vi "Iterator.vi"(8 "error in":errorcluster, 11 "Iterator Actor in":refnum<class "Abstract Iterator Actor.lvclass">) -> (0 "error out":errorcluster, 3 "Iterator Actor out":refnum<class "Abstract Iterator Actor.lvclass">)   [LabVIEW 2023, in "Iterator Actor.lvlib" / "Abstract Iterator Actor.lvclass"]
doc: "(<B>Filename</B>: Actor Framework.lvlib:Actor.lvclass:Actor Core.vi)\n\nReceives messages to the actor, reacts to them, and initiates any error handling that may shut the actor down.\n\nDescendant classes may override this VI to append parallel tasks for the actor to complete while it handles messages. Overrides use the Call Parent Method node."
uses:
  Abstract Iterator Actor.lvclass
  Abstract Iterator Actor.lvclass/Abstract Iterator Actor.ctl
  <vilib>/ActorFramework/Actor/Actor.lvclass/Actor.ctl
  <vilib>/ActorFramework/Message Enqueuer/Message Enqueuer.lvclass/Message Enqueuer.ctl
  Stop Reason.ctl
  <vilib>/ActorFramework/Message Enqueuer/Init from Existing Queue.vi
  <vilib>/ActorFramework/Message Enqueuer/Message Enqueuer.lvclass
  <vilib>/ActorFramework/Actor/Actor.lvclass
  Iterator Actor/Iterator Actor Messages/Report Iterations End Msg/Report Iterations End Msg.lvclass
  Iterator Actor/Iterator Actor Messages/Write Stop Reason Msg/Write Stop Reason Msg.lvclass
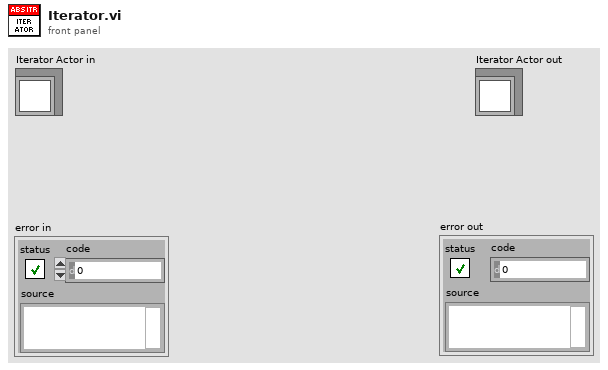
[diagram p1: front panel]
types:
  T1 = typedef "Iterator Actor.lvlib/Abstract Iterator Actor.lvclass/Iterator Settings.ctl" = cluster{"Prepare timeout (ms)":i32, "Iterate timeout (ms)":i32, "Conclude timeout (ms)":i32, "Iterate period (ms)":i32, "Number of iterations":i32, "Time before stop (ms)":i32, "Active Stop Conditions":T2, "Prepare Msg":refnum<class "Message.lvclass">, "Iterate Msg":refnum<class "Message.lvclass">, "Conclude Msg":refnum<class "Message.lvclass">, "Iterations End Report":refnum<class "Iterator Report Iterations End Msg.lvclass">}
  T2 = typedef "Iterator Actor.lvlib/Abstract Iterator Actor.lvclass/Active Stop Conditions.ctl" = cluster{"Number of Iterations":bool, "Time Elapsed":bool, "Iteration Result":bool}
  T3 = typedef "Iterator Actor.lvlib/Abstract Iterator Actor.lvclass/Stop Reason.ctl" = enum16{"Number of Iterations", "Time Elapsed", "Stopped Internally", "Stopped Externally"}
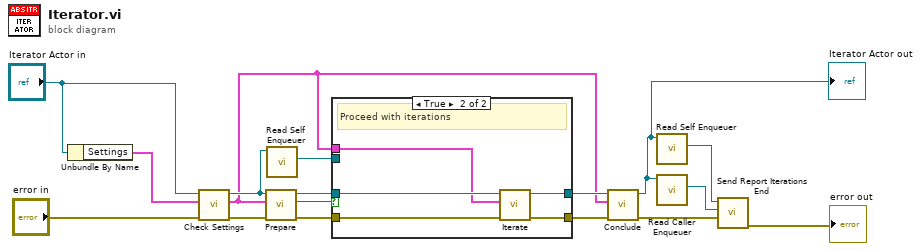
[diagram p0: block diagram]
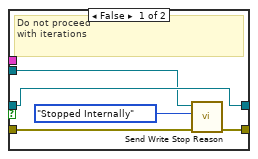
[diagram p2: hidden frame]
diagram:
  n1 = Unbundle By Name("Iterator Actor in") -> ("Settings"=w1:T1)
  n2 = call-dynamic "Check Settings.vi"("error in (no error)"="error in", "Iterator Settings in"=w1, "Abstract Iterator Actor in"="Iterator Actor in") -> ("error out"=w12:errorcluster, "Iterator Settings out"=w6:T1, "Abstract Iterator Actor out"=w7:refnum<class "Abstract Iterator Actor.lvclass">)  [unwired: 6 in]
  n3 = call-dynamic "Prepare.vi"("error in"=w12, "Iterator Settings"=w6, "Abstract Iterator Actor in"=w7) -> ("error out"=w13:errorcluster, "Reply"=w14:bool, "Abstract Iterator Actor out"=w16:refnum<class "Abstract Iterator Actor.lvclass">)  [unwired: 6 in]
  n4 = call <vilib>:"Read Self Enqueuer.vi"("Actor"=w7) -> ("Self Enqueuer"=w9:refnum<class "Message Enqueuer.lvclass">)  [unwired: 10 in]
  n5 = case shown="True" w14 {
    tunnel: [w20 w27] -> w17
    tunnel: w6 -> [_ w23]
    tunnel: w16 -> [w22 w26]
    tunnel: [w22 w25] -> w15
    tunnel: w13 -> [w21 w24]
    tunnel: w9 -> [w19 _]
    frame False {
      # "Do not proceed \nwith iterations"
      n6 = call "Send Write Stop Reason.vi"("error in (no error)"=w21, "Stop Reason"=Stop_Reason."Stopped Internally", "Message Enqueuer in"=w19) -> ("error out"=w20:errorcluster)  [unwired: 7 in, 1 out]
    }
    frame True {
      # "Proceed with iterations"
      n7 = call-dynamic "Iterate.vi"("error in (no error)"=w24, "Iterator Settings"=w23, "Abstract Iterator Actor in"=w26) -> ("error out"=w27:errorcluster, "Abstract Iterator Actor out"=w25:refnum<class "Abstract Iterator Actor.lvclass">)  [unwired: 7 in]
    }
  }
  n8 = call-dynamic "Conclude.vi"("error in (no error)"=w17, "Iterator Settings"=w6, "Abstract Iterator Actor in"=w15) -> ("error out"=w11:errorcluster, "Abstract Iterator Actor out"=w4:refnum<class "Abstract Iterator Actor.lvclass">)  [unwired: 7 in]
  "Iterator Actor out" <- w4
  n9 = call <vilib>:"Read Self Enqueuer.vi"("Actor"=w4) -> ("Self Enqueuer"=w8:refnum<class "Message Enqueuer.lvclass">)  [unwired: 10 in]
  n10 = call <vilib>:"Read Caller Enqueuer.vi"("Actor"=w4) -> ("Caller Enqueuer"=w10:refnum<class "Message Enqueuer.lvclass">)  [unwired: 10 in]
  n11 = call "Send Report Iterations End.vi"("Iterator Error"=w11, "Caller Enqueuer in"=w10, "Message Enqueuer in"=w8) -> ("error out"=→"error out":errorcluster)  [unwired: 7 in, 1 out]
